vi "Autonomous Independent.vi"() -> ()   [LabVIEW 2016]
doc: "This VI is called when autonomous begins, and will automatically be terminated when autonomous ends. You can carry out timed or sensor driven robot movement independently without needing to return to the caller."
uses:
  <vilib>/Rock Robotics/Network Tables/NT Read String.vi
  Robot Global Data.vi
  <vilib>/Rock Robotics/WPI/Utilities/WPI_GetSetVariantRefNum.vi
  <vilib>/addons/control/pid/pid.llb/PID (DBL).vi
  <vilib>/Rock Robotics/WPI/RobotDrive/WPI_RobotDriveArcadeDrive_Standard(NoSaturation).vi
  <vilib>/Rock Robotics/Network Tables/NT Write Numeric Array.vi
  <vilib>/addons/control/pid/NI_PID_pid.lvlib
panel:
  in  "PID gains L":T1={"proportional gain (Kc)"=1.5e-05, "integral time (Ti, min)"=1e-07, "derivative time (Td, min)"=0.0} {"derivative time (Td, min)" format="%.3f"; "integral time (Ti, min)" format="%.6f"; "proportional gain (Kc)" format="%.6f"}
  in  "PID gains R":T1={"proportional gain (Kc)"=1.5e-05, "integral time (Ti, min)"=1e-07, "derivative time (Td, min)"=0.0} {"derivative time (Td, min)" format="%.3f"; "integral time (Ti, min)" format="%.6f"; "proportional gain (Kc)" format="%.6f"}
  in  "Range":cluster{"output high":dbl, "output low":dbl}={"output high"=1.0, "output low"=-1.0} {"output low" format="%.2f"; "output high" format="%.2f"}
  out "Right V":cluster{"output":dbl, dbl, "Numeric":dbl}(graph)
  out "Left V":cluster{"output":dbl, dbl, "Numeric":dbl}(graph)
  in  "Speed":dbl=0.5 format="%#_13g"
  out "Current Movement, for debugging":T2 {"Y Joystick Value" scale=1.0..-1.0; "X Joystick Value" scale=-1.0..1.0}
  in  "Array of robot movements":T3(array[cluster])=[{"X Joystick Value"=0.39393939393939403, "Y Joystick Value"=0.0, "Delay (sec)"=1.0, "Movement Name"="turn"}, {"X Joystick Value"=-0.3737373737373737, "Y Joystick Value"=0.0, "Delay (sec)"=1.0, "Movement Name"="turn back"}] {"Y Joystick Value" scale=1.0..-1.0; "X Joystick Value" scale=-1.0..1.0}
  # "Be sure to right-click and choose Data Operations>>Make Current Value default if you want to save the array values with the VI"
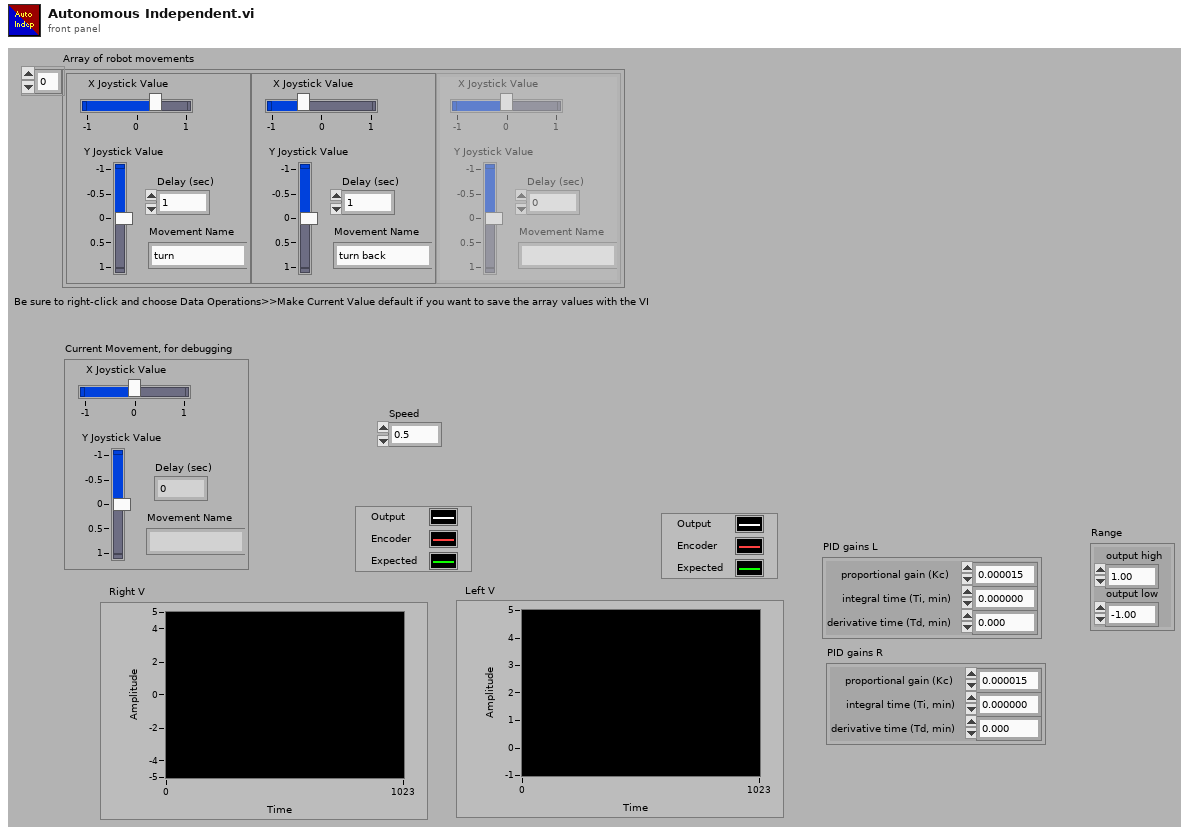
[diagram p1: front panel]
types:
  T1 = cluster{"proportional gain (Kc)":dbl, "integral time (Ti, min)":dbl, "derivative time (Td, min)":dbl}
  T2 = cluster{"X Joystick Value":dbl, "Y Joystick Value":dbl, "Delay (sec)":dbl, "Movement Name":string}
  T3 = cluster{"X Joystick Value":dbl, "Y Joystick Value":dbl, "Delay (sec)":dbl, "Movement Name":string}[]
  T4 = typedef "WPI_RobotDriveDevRef.ctl" = cluster{"DevStatus":errorcluster, "Motors[]":T5[], "Square Inputs":bool, "Max Output":dbl}
  T5 = typedef "WPI_MotorControlDeviceRef.ctl" = cluster{"DeviceStatus":errorcluster, "Type":T6, "PWM":cluster{"PWM Channel":T7, "DeadBand":T8}, "CAN":cluster{"Device Number":u8, "SetOutput VI Ref":variant, "GetOutput VI Ref":variant, "Enable VI Ref":variant, "Disable VI Ref":variant, "Data":variant}, "Invert":bool}
  T6 = typedef "WPI_MotorControlType.ctl" = enum16{"PWM", "CAN"}
  T7 = typedef "FPGA_DIOPWMChannel.ctl" = enum8{"PWM 0", "PWM 1", "PWM 2", "PWM 3", "PWM 4", "PWM 5", "PWM 6", "PWM 7", "PWM 8", "PWM 9", "PWM MXP 0", "PWM MXP 1", "PWM MXP 2", "PWM MXP 3", "PWM MXP 4", "PWM MXP 5", "PWM MXP 6", "PWM MXP 7", "PWM MXP 8", "PWM MXP 9", "Invalid"}
  T8 = typedef "WPI_PWMDeadband.ctl" = cluster{"Name":string, "maxPositivePwm":i32, "minPositivePwm":i32, "centerPwm":i32, "maxNegativePwm":i32, "minNegativePwm":i32, "angularRange":u16}
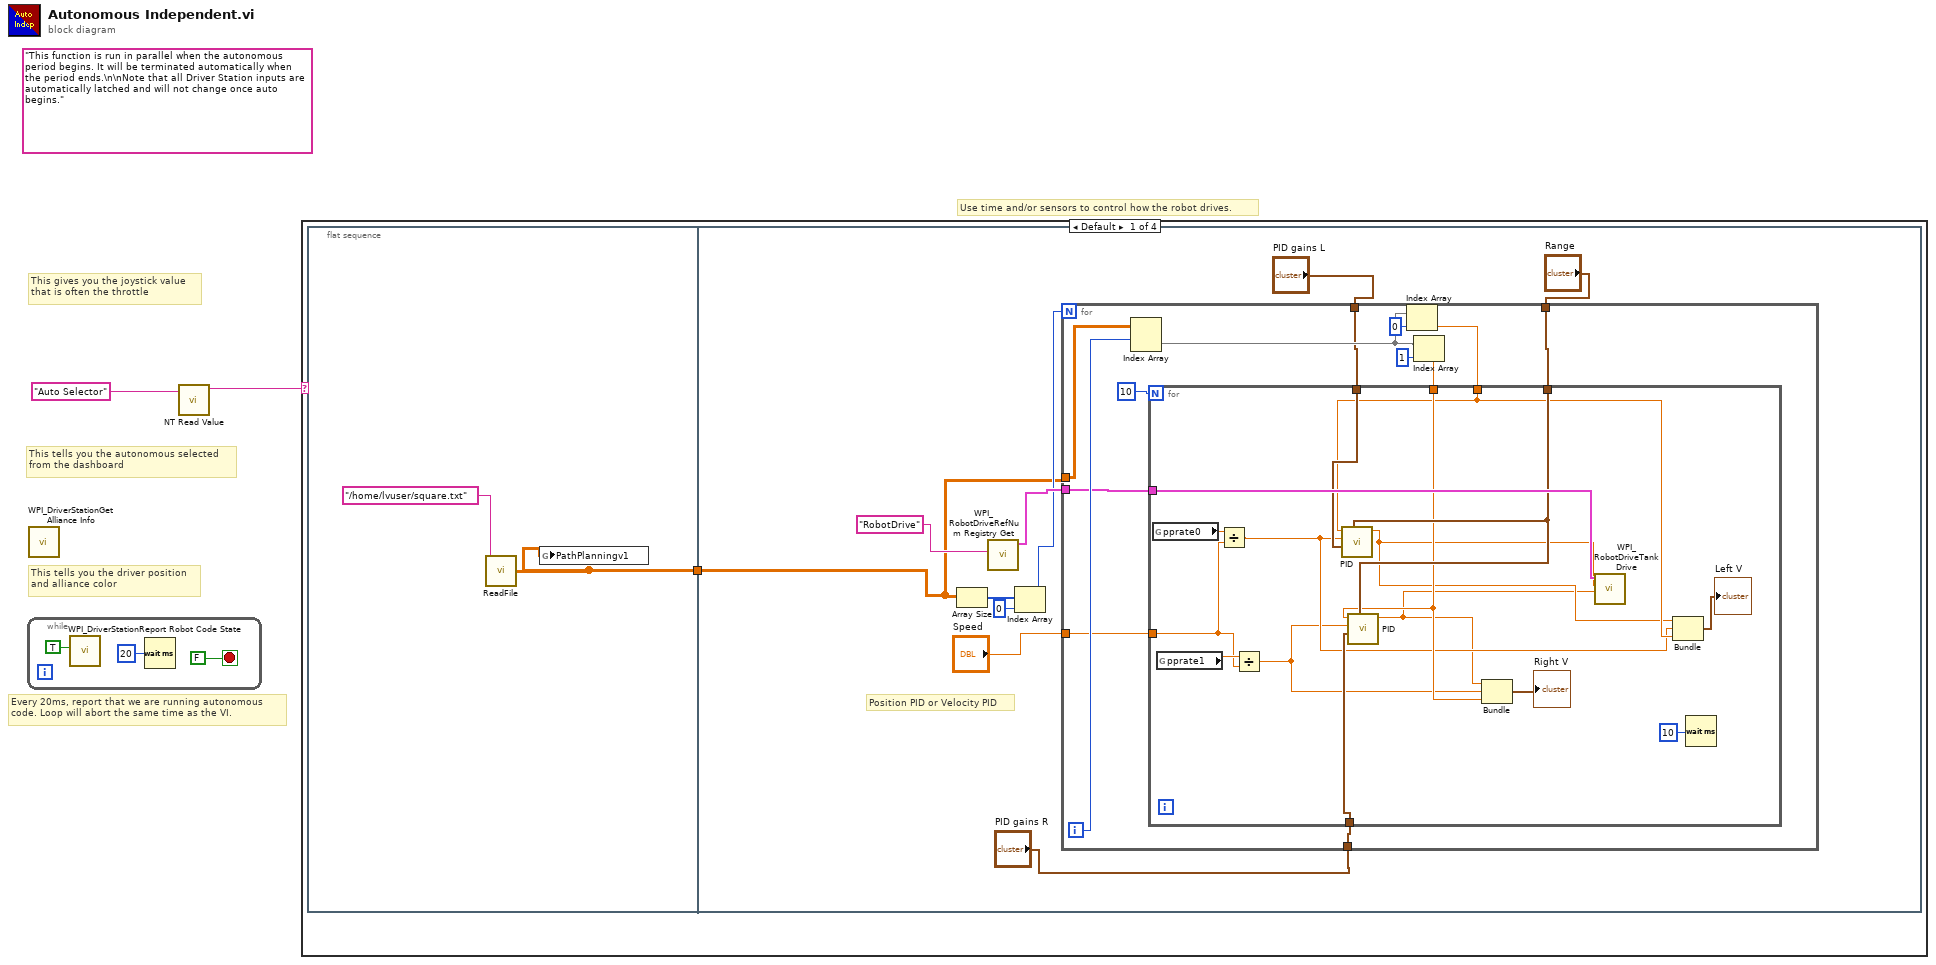
[diagram p0: block diagram]
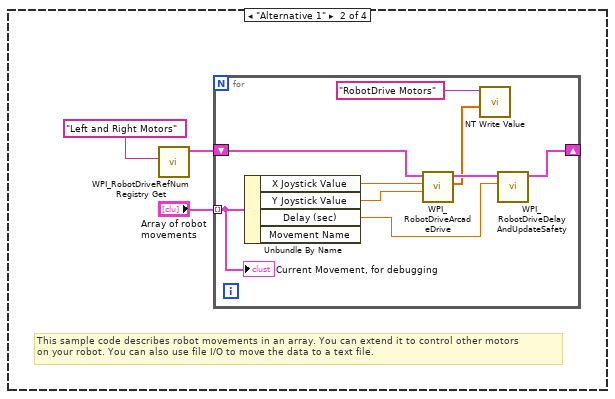
[diagram p2: hidden frame]
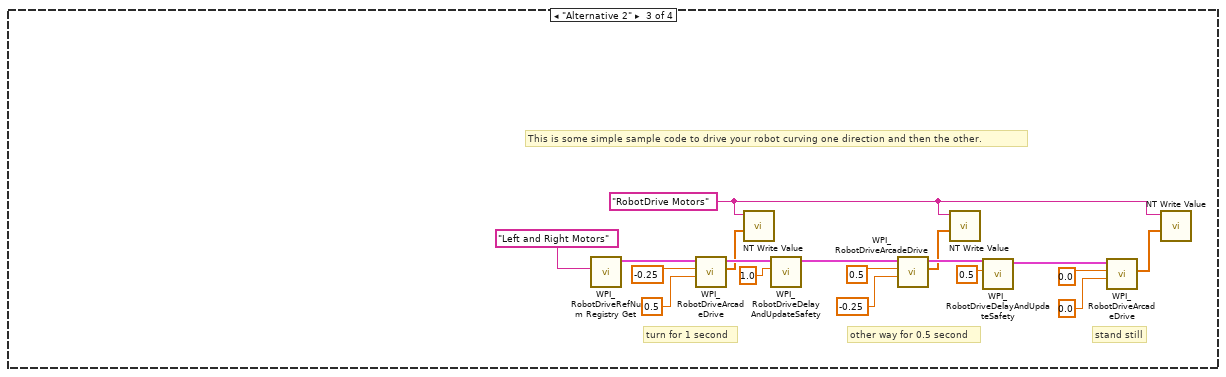
[diagram p3: hidden frame]
diagram:
  (unwired) "This function is run in parallel when the autonomous period begins. It will be terminated automatically when the period ends.\n\nNote that all Driver Station inputs are automatically latched and will not change once auto begins."
  # "This tells you the autonomous selected\nfrom the dashboard"
  # "Every 20ms, report that we are running autonomous\ncode. Loop will abort the same time as the VI."
  # "This gives you the joystick value\nthat is often the throttle"
  # "Use time and/or sensors to control how the robot drives."
  # "This tells you the driver position\nand alliance color"
  n1 = while {
    stop <- FALSE stop-if-true
    n2 = call <vilib>:"WPI_DriverStationReport Robot Code State.vi"("Autonomous"=TRUE) -> ()  [unwired: 10 in, 1 out]
    n3 = Wait (ms)(milliseconds to wait=u32 20) -> ()  [unwired: 1 out]
  }
  n4 = call <vilib>:"WPI_DriverStationGet Alliance Info.vi"() -> ()  [unwired: 12 out]
  n5 = call-poly <vilib>:"NT Read Value.vi"("Name"="Auto Selector") -> ("String"=w1:string)  [unwired: 9 in, 1 out]
  n6 = case shown="Default" w1 {
    frame Default {
      n7 = flat-sequence {
        tunnel: [w7] -> w6
        tunnel: w6 -> [w10]
        frame #0 {
          n8 = call "ReadFile.vi"("Name"="/home/lvuser/square.txt") -> ("Array - Numeric"=w7:dbl[][])
          n9 = global write "Robot Global Data.vi" "PathPlanningv1"(w7) -> ()
        }
        frame #1 {
          # "Position PID or Velocity PID"
          n10 = Array Size(array=w10) -> (size(s)=w18:i32[])
          n11 = call <vilib>:"WPI_RobotDriveRefNum Registry Get.vi"("refnum name"="RobotDrive") -> ("RobotDriveDevRef"=w15:T4)  [unwired: 9 in, 1 out]
          n12 = Index Array(array=w18, index=0) -> (element=w14:i32)
          n13 = for {
            N: w14 -> [_]
            tunnel: w10 -> [w28]
            tunnel: "PID gains R" -> [w23]
            tunnel: "PID gains L" -> [w22]
            tunnel: "Range" -> [w21]
            tunnel: w15 -> [w20]
            tunnel: "Speed" -> [w19]
            i -> [w25]
            n14 = Index Array(array=w28, index (row)=w25) -> (element=w31:dbl[])  [unwired: 1 in]
            n15 = Index Array(array=w31, index=0) -> (element=w27:dbl)
            n16 = Index Array(array=w31, index=1) -> (element=w26:dbl)
            n17 = for {
              N: 10 -> [_]
              tunnel: w27 -> [w41]
              tunnel: w26 -> [w42]
              tunnel: w23 -> [w45]
              tunnel: w22 -> [w44]
              tunnel: w21 -> [w43]
              tunnel: w20 -> [w46]
              tunnel: w19 -> [w34]
              n18 = global read "Robot Global Data.vi" "pprate0"() -> (w38:dbl)
              n19 = global read "Robot Global Data.vi" "pprate1"() -> (w35:dbl)
              n20 = Divide(x=w38, y=w34) -> (x/y=w37:dbl)
              n21 = Divide(x=w35, y=w34) -> (x/y=w36:dbl)
              n22 = call-poly <vilib>:"PID.vi"("output range"=w43, "PID gains"=w44, "process variable"=w37, "setpoint"=w41) -> ("output"=w33:dbl)  [unwired: 6 in, 1 out]
              n23 = call-poly <vilib>:"PID.vi"("output range"=w43, "PID gains"=w45, "process variable"=w36, "setpoint"=w42) -> ("output"=w32:dbl)  [unwired: 6 in, 1 out]
              n24 = Bundle("output"=w32, w36, "Numeric"=w42) -> (→"Right V":cluster{"output":dbl, dbl, "Numeric":dbl})  [unwired: 1 in]
              n25 = call <vilib>:"WPI_RobotDriveTankDrive.vi"("Right axis value"=w32, "Left axis value"=w33, "RobotDriveDevRef"=w46) -> ()  [unwired: 6 in, 3 out]
              n26 = Bundle("output"=w33, w37, "Numeric"=w41) -> (→"Left V":cluster{"output":dbl, dbl, "Numeric":dbl})  [unwired: 1 in]
              n27 = Wait (ms)(milliseconds to wait=10) -> ()  [unwired: 1 out]
            }
          }
        }
      }
    }
    frame "Alternative 1" {
      # "This sample code describes robot movements in an array. You can extend it to control other motors\non your robot. You can also use file I/O to move the data to a text file."
      n28 = call <vilib>:"WPI_RobotDriveRefNum Registry Get.vi"("refnum name"="Left and Right Motors") -> ("RobotDriveDevRef"=w49:T4)  [unwired: 1 in, 9 out]
      n29 = for {
        shift-right: [w57] -> _
        shift-left: w49 -> [w58]
        tunnel: "Array of robot movements" -> [w53] mode=indexing
        n30 = Unbundle By Name(w53) -> ("X Joystick Value"=w56:dbl, "Y Joystick Value"=w55:dbl, "Delay (sec)"=w54:dbl)  [unwired: 1 out]
        n31 = call-poly <vilib>:"WPI_RobotDriveArcadeDrive.vi"("Y axis value"=w55, "X axis value"=w56, "RobotDriveDevRef"=w58) -> ("Motor Values"=w51:dbl[], "RobotDriveDevRef"=w59:T4)  [unwired: 1 in, 6 out]
        n32 = call-poly <vilib>:"NT Write Value.vi"("Numeric Array"=w51, "Name"="RobotDrive Motors") -> ()  [unwired: 9 in, 1 out]
        n33 = call <vilib>:"WPI_RobotDriveDelayAndUpdateSafety.vi"("Delay (s)"=w54, "RobotDriveDevRef"=w59) -> ("RobotDriveDevRef 2"=w57:T4)  [unwired: 8 in, 1 out]
        "Current Movement, for debugging" <- w53
      }
    }
    frame "Alternative 2" {
      w61 = "RobotDrive Motors" ("Name")
      # "This is some simple sample code to drive your robot curving one direction and then the other."
      # "stand still"
      # "other way for 0.5 second"
      # "turn for 1 second"
      n34 = call <vilib>:"WPI_RobotDriveRefNum Registry Get.vi"("refnum name"="Left and Right Motors") -> ("RobotDriveDevRef"=w77:T4)  [unwired: 1 in, 9 out]
      n35 = call-poly <vilib>:"WPI_RobotDriveArcadeDrive.vi"("Y axis value"=0.5 ("X axis value"), "X axis value"=-0.25, "RobotDriveDevRef"=w77) -> ("Motor Values"=w60:dbl[], "RobotDriveDevRef"=w70:T4)  [unwired: 1 in, 6 out]
      n36 = call-poly <vilib>:"NT Write Value.vi"("Numeric Array"=w60, "Name"=w61) -> ()  [unwired: 9 in, 1 out]
      n37 = call <vilib>:"WPI_RobotDriveDelayAndUpdateSafety.vi"("Delay (s)"=1.0, "RobotDriveDevRef"=w70) -> ("RobotDriveDevRef 2"=w71:T4)  [unwired: 8 in, 1 out]
      n38 = call-poly <vilib>:"WPI_RobotDriveArcadeDrive.vi"("Y axis value"=-0.25 ("X axis value"), "X axis value"=0.5, "RobotDriveDevRef"=w71) -> ("Motor Values"=w62:dbl[], "RobotDriveDevRef"=w72:T4)  [unwired: 1 in, 6 out]
      n39 = call-poly <vilib>:"NT Write Value.vi"("Numeric Array"=w62, "Name"=w61) -> ()  [unwired: 9 in, 1 out]
      n40 = call <vilib>:"WPI_RobotDriveDelayAndUpdateSafety.vi"("Delay (s)"=0.5, "RobotDriveDevRef"=w72) -> ("RobotDriveDevRef 2"=w73:T4)  [unwired: 8 in, 1 out]
      n41 = call-poly <vilib>:"WPI_RobotDriveArcadeDrive.vi"("Y axis value"=0.0 ("X axis value"), "X axis value"=0.0, "RobotDriveDevRef"=w73) -> ("Motor Values"=w63:dbl[])  [unwired: 1 in, 7 out]
      n42 = call-poly <vilib>:"NT Write Value.vi"("Numeric Array"=w63, "Name"=w61) -> ()  [unwired: 9 in, 1 out]
    }
    frame "Your Turn" {
    }
  }
